vi "Enable PreAmp.vi"(0 "VISA resource name":refnum<visa-resource-name>, 5 "Enable PreAmp (F:Disable)":bool, 11 "error in (no error)":errorcluster) -> (4 "VISA resource name out":refnum<visa-resource-name>, 15 "error out":errorcluster)   [LabVIEW 2023, in "Anritsu Signal Analyzer Series.lvlib"]
doc: "Enables Preamp"
uses:
  Anritsu Signal Analyzer Series.lvlib
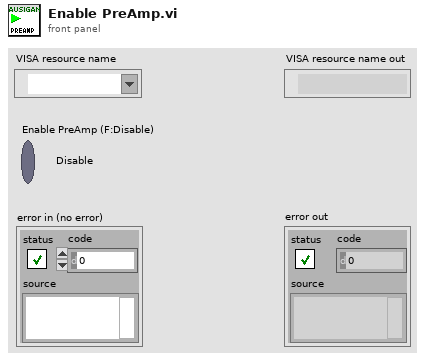
[diagram p1: front panel]
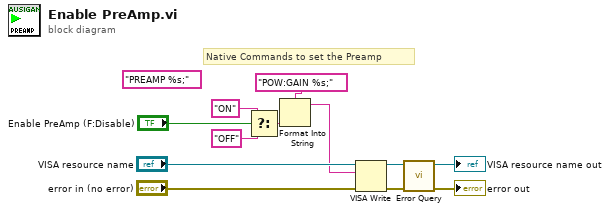
[diagram p0: block diagram]
diagram:
  (unwired) "PREAMP %s;" ("_CommandSet")
  # "Native Commands to set the Preamp"
  n1 = Select(t="ON", s="Enable PreAmp (F:Disable)", f="OFF") -> (s? t:f=w2:string)
  n2 = Format Into String(format string="POW:GAIN %s;" ("_CommandSet"), w2) -> (resulting string=w1:string)  [unwired: 2 in, 1 out]
  n3 = VISA Write(VISA resource name="VISA resource name", write buffer=w1, error in (no error)="error in (no error)") -> (VISA resource name out=w8:refnum<visa-resource-name>, error out=w7:errorcluster)  [unwired: 1 out]
  n4 = call "Error Query.vi"("error in (no error)"=w7, "VISA resource name"=w8) -> ("error out"=→"error out":errorcluster, "VISA resource name out"=→"VISA resource name out":refnum<visa-resource-name>)  [unwired: 6 in, 2 out]
